vi "Read Message (Serial).vi"(8 "error in":errorcluster, 9 "options":T2={"ignore timeout error"=TRUE, "timeout ms (1000)"=1000}, 11 "connection info in":T4) -> (0 "error out":errorcluster, 1 "name":T3, 2 "data string":string, 3 "connection info out":T4, 4 "data info":T1, 5 "timed out?":bool)   [LabVIEW 2013, in "NI STM.lvlib"]
doc: "This VI reads an incoming package of data from a host. This VI parses the package and extracts the data name and type as described in the meta data.\n\nFor the package to be parsed correctly, the meta data must be consistent in both the sender and the receiver. The data is packaged based on the existing meta data on the sender. \n\nUse the \"STM Read Meta Data\" and \"STM Write Meta Data\" VIs to ensure that both client and server have the same meta data.\n\nThe data is returned as a string. It is the responsibility of the user to cast it to the appropriate type."
uses:
  NI STM.lvlib
  Serial Connection Info.ctl
  SubVIs/MetaDataElement.ctl
  Serial Read Options.ctl
  Serial Data Info.ctl
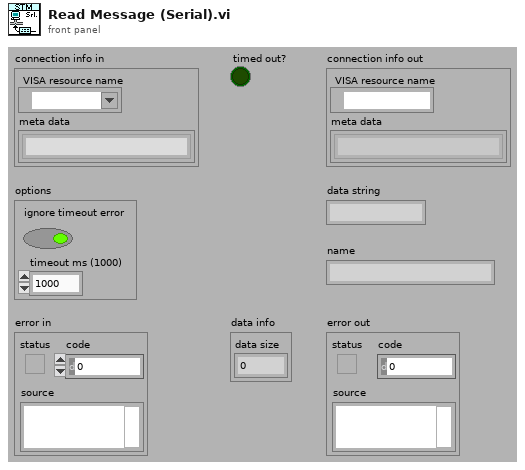
[diagram p1: front panel]
types:
  T1 = typedef "NI STM.lvlib/Serial Data Info.ctl" = cluster{"data size":u32}
  T2 = typedef "NI STM.lvlib/Serial Read Options.ctl" = cluster{"ignore timeout error":bool, "timeout ms (1000)":u32}
  T3 = typedef "NI STM.lvlib/MetaDataElement.ctl" = string
  T4 = typedef "NI STM.lvlib/Serial Connection Info.ctl" = cluster{"VISA resource name":refnum<visa-resource-name>, "meta data":T3[]}
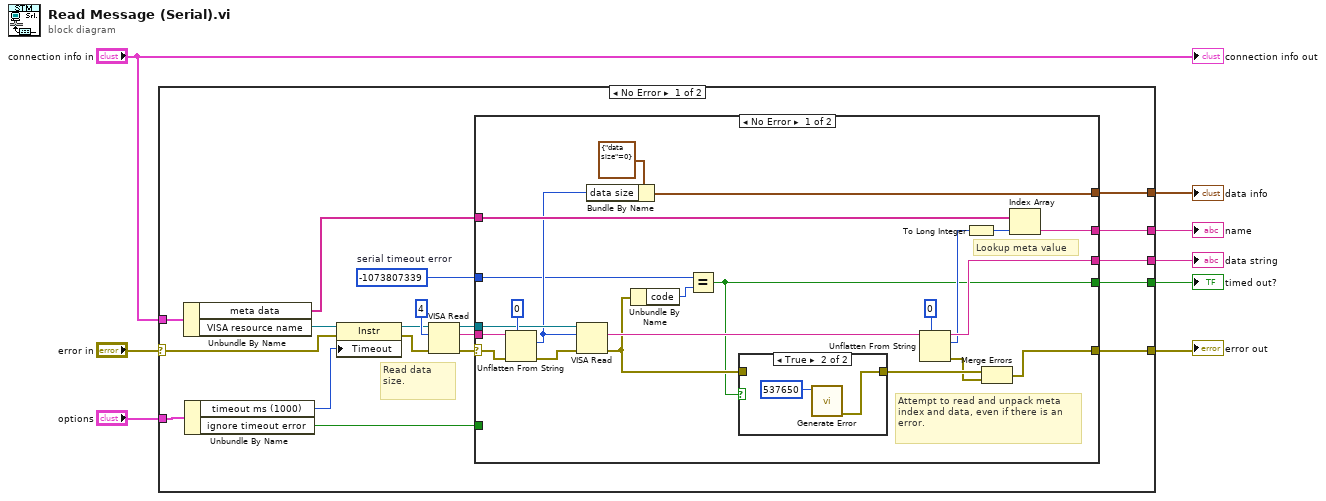
[diagram p0: block diagram]
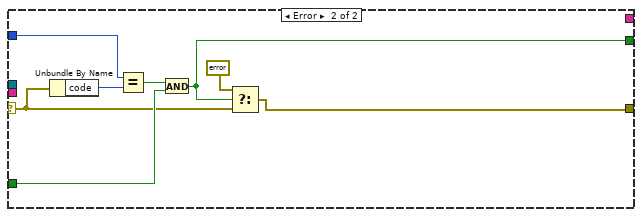
[diagram p3: hidden frame]
diagram:
  n1 = case shown="No Error" "error in" {
    selector: "error in" -> [w13 w61]
    tunnel: "connection info in" -> [w10 _]
    tunnel: [w23 w61] -> w8
    tunnel: [w22 _] -> w7
    tunnel: [w21 _] -> w6
    tunnel: [w20 _] -> w5
    tunnel: [w19 _] -> w2
    tunnel: "options" -> [w16 _]
    frame No Error {
      w9 = -1073807339  # serial timeout error
      # "Read data size."
      n2 = Unbundle By Name(w10) -> ("meta data"=w17:T3[], "VISA resource name"=w15:refnum<visa-resource-name>)
      n3 = Unbundle By Name(w16) -> ("timeout ms (1000)"=w14:u32, "ignore timeout error"=w18:bool)
      n4 = property class="Instr"(reference=w15, error in=w13, "Timeout"=w14) -> (reference out=w11:refnum<visa-resource-name>, error out=w12:errorcluster)
      n5 = VISA Read(VISA resource name=w11, byte count=u32 4 ("bytes to read"), error in (no error)=w12) -> (VISA resource name out=w25:refnum<visa-resource-name>, read buffer=w26:string, error out=w24:errorcluster)  [unwired: 1 out]
      n6 = case shown="No Error" w24 {
        selector: w24 -> [w45 w53]
        tunnel: w26 -> [w46 _]
        tunnel: w25 -> [w48 _]
        tunnel: w17 -> [w47 _]
        tunnel: [w28 w56] -> w23
        tunnel: w18 -> [_ w55]
        tunnel: [w31 w54] -> w22
        tunnel: [w44 _] -> w21
        tunnel: [w40 _] -> w20
        tunnel: [w36 _] -> w19
        tunnel: w9 -> [w34 w57]
        frame No Error {
          # "Attempt to read and unpack meta index and data, even if there is an error."
          # "Lookup meta value"
          n7 = Unflatten From String(type=u32 0 ("bytes to read"), binary string=w46, error in (no error)=w45) -> (value=w37:u32, error out=w42:errorcluster)  [unwired: 1 in, 2 out]
          n8 = VISA Read(VISA resource name=w48, byte count=w37, error in (no error)=w42) -> (read buffer=w43:string, error out=w32:errorcluster)  [unwired: 2 out]
          n9 = Bundle By Name(cluster=T1 {"data size"=0} ("Data Info"), "data size"=w37) -> (w36:T1)
          n10 = Unbundle By Name(w32) -> ("code"=w33:i32)
          n11 = Equal?(x=w34, y=w33) -> (x = y?=w31:bool)
          n12 = case shown="True" w31 {
            tunnel: w32 -> [w50 _]
            tunnel: [w50 w51] -> w30
            frame False {
            }
            frame True {
              n13 = call "Generate Error.vi"("code"=537650) -> ("error out"=w51:errorcluster)  [unwired: 10 in]
            }
          }
          n14 = Unflatten From String(type=u16 0 ("bytes to read"), binary string=w43) -> (rest of the binary string=w40:string, value=w38:u16, error out=w29:errorcluster)  [unwired: 1 in, 2 out]
          n15 = To Long Integer(number=w38) -> (32bit integer=w39:i32)
          n16 = Merge Errors(w30, w29) -> (w28:errorcluster)
          n17 = Index Array(array=w47, index=w39) -> (element=w44:T3)
        }
        frame Error {
          n18 = Unbundle By Name(w53) -> ("code"=w58:i32)
          n19 = Equal?(x=w57, y=w58) -> (x = y?=w60:bool)
          n20 = And(x=w60, y=w55) -> (x .and. y?=w54:bool)
          n21 = Select(t=errorcluster {"status"=FALSE, "code"=0, "source"=""} ("error out"), s=w54, f=w53) -> (s? t:f=w56:errorcluster)
        }
      }
    }
    frame Error {
    }
  }
  "error out" <- w8
  "timed out?" <- w7
  "data string" <- w5
  "name" <- w6
  "data info" <- w2
  "connection info out" <- "connection info in"
